vi "Actor Core.vi"(8 "error in":errorcluster, 11 "Nested in":refnum<class "UI Actor.lvclass">) -> (0 "error out":errorcluster, 3 "Actor out":refnum<class "Actor.lvclass">)   [LabVIEW 2020, in "UI Actor.lvlib" / "UI Actor.lvclass"]
doc: "(<B>Filename</B>: Actor Framework.lvlib:Actor.lvclass:Actor Core.vi)\n\nReceives messages to the actor, reacts to them, and initiates any error handling that may shut the actor down.\n\nDescendant classes may override this VI to append parallel tasks for the actor to complete while it handles messages. Overrides use the Call Parent Method node."
uses:
  UI Actor.lvclass
  C:/Program Files (x86)/National Instruments/LabVIEW 2020/vi.lib/ActorFramework/Actor/Actor.lvclass
  <vilib>/ActorFramework/Actor/Actor.lvclass
  <vilib>/ActorFramework/Actor/Actor.lvclass/Actor.ctl
  <vilib>/ActorFramework/Message Enqueuer/Message Enqueuer.lvclass/Message Enqueuer.ctl
  UI Actor.lvclass/UI Actor.ctl
  UI Actor Messages/Read ADC Msg/Read ADC Msg.lvclass/Read ADC Msg.ctl
  UI Actor Messages/Set Pin Status Msg/Set Pin Status Msg.lvclass/Set Pin Status Msg.ctl
  <vilib>/ActorFramework/Message Enqueuer/Init from Existing Queue.vi
  <vilib>/ActorFramework/Message Enqueuer/Enqueue.vi
  <vilib>/ActorFramework/Stop Msg/Stop Msg.lvclass
  C:/Program Files (x86)/National Instruments/LabVIEW 2020/vi.lib/ActorFramework/Message/Message.lvclass
  UI Actor Messages/Read ADC Msg/Read ADC Msg.lvclass
  UI Actor Messages/Set Pin Status Msg/Set Pin Status Msg.lvclass
  <vilib>/ActorFramework/Message Priority Queue/Priority Enqueue.vi
  <vilib>/ActorFramework/Message Enqueuer/Message Enqueuer.lvclass
  UI Actor Messages/Set Port Status Msg/Set Port Status Msg.lvclass
panel:
  out "Port Leds":bool[](array[boolean])
  in  "Port Value":string
  in  "Set Port Status":bool
  in  "Port":string(combo)
  out "Boolean 8":bool
  out "Boolean 7":bool
  out "Boolean 6":bool
  out "Boolean 5":bool
  out "Boolean 4":bool
  out "Boolean 3":bool
  out "Boolean 2":bool
  out "Boolean":bool
  out "Array":bool[](array[boolean])
  in  "Value":string(combo)
  in  "Set Pin Status":bool
  in  "Pin LED":string(combo)
  in  "Canal LED":string(combo)
  out "TERMINAL READING":string
  in  "Canal ADC":string(combo)
  in  "Read ADC":bool
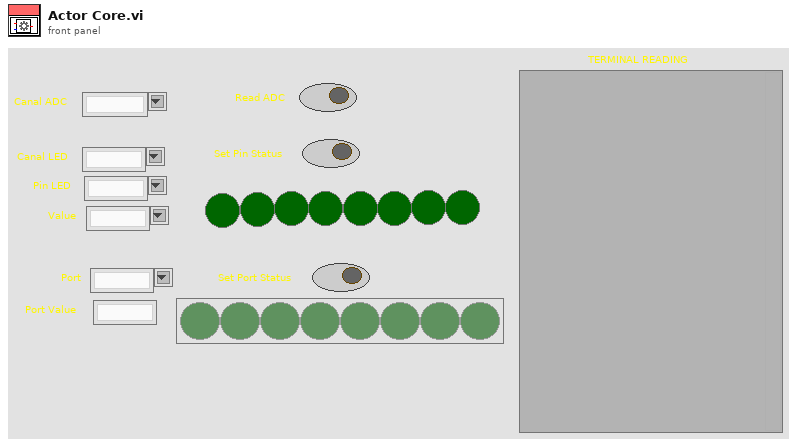
[diagram p1: front panel]
types:
  T1 = cluster{"Stop":refnum<user-event>, "TERMINAL READING":refnum<user-event>, "Array":refnum<user-event>, "Boolean 2":refnum<user-event>, "Boolean 3":refnum<user-event>, "Boolean 6":refnum<user-event>, "Boolean 8":refnum<user-event>, "Boolean 4":refnum<user-event>, "Boolean":refnum<user-event>, "Boolean 5":refnum<user-event>, "Boolean 7":refnum<user-event>, "Port Leds":refnum<user-event>}
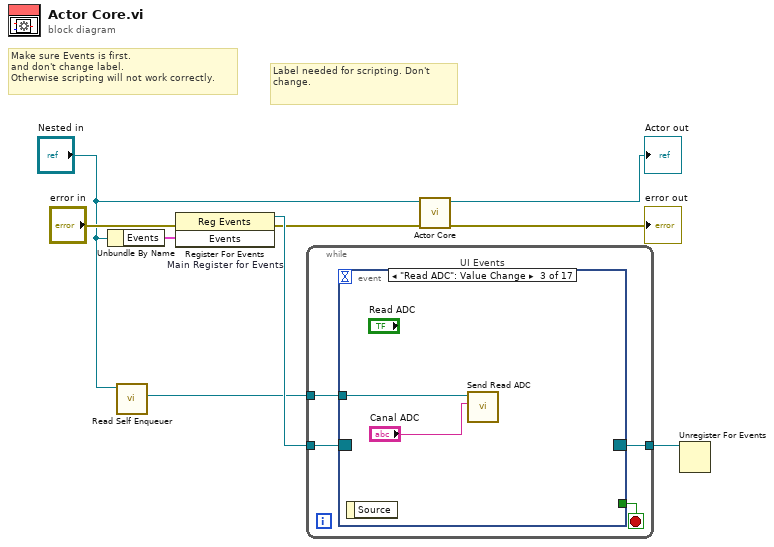
[diagram p0: block diagram]
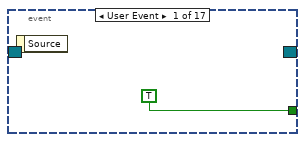
[diagram p2: hidden frame]
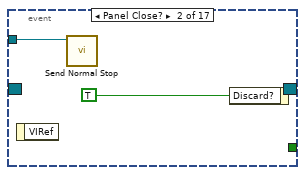
[diagram p3: hidden frame]
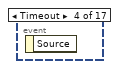
[diagram p4: hidden frame]
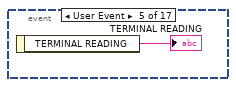
[diagram p5: hidden frame]
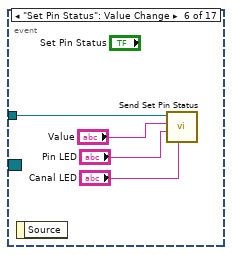
[diagram p6: hidden frame]
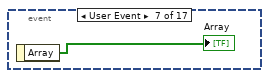
[diagram p7: hidden frame]
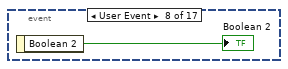
[diagram p8: hidden frame]
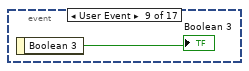
[diagram p9: hidden frame]
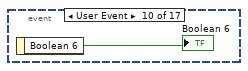
[diagram p10: hidden frame]
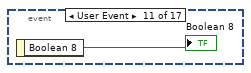
[diagram p11: hidden frame]
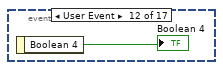
[diagram p12: hidden frame]
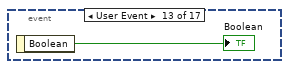
[diagram p13: hidden frame]
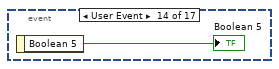
[diagram p14: hidden frame]
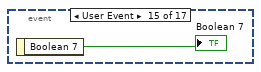
[diagram p15: hidden frame]
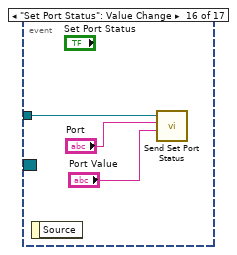
[diagram p16: hidden frame]
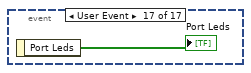
[diagram p17: hidden frame]
diagram:
  # "Label needed for scripting. Don't change."
  # "Make sure Events is first.\nand don't change label.\nOtherwise scripting will not work correctly."
  n1 = Unbundle By Name("Nested in") -> ("Events"=w6:T1)
  n2 = call <vilib>:"Read Self Enqueuer.vi"("Actor"="Nested in") -> ("Self Enqueuer"=w4:refnum<class "Message Enqueuer.lvclass">)  [unwired: 10 in]
  n3 = register-events "Main Register for Events"(error in="error in", w6) -> (reference out=w7:refnum<event-registration>, error out=w2:errorcluster)  [unwired: 1 in]
  n4 = while {
    tunnel: w7 -> [w13]
    tunnel: [w11] -> w5
    tunnel: w4 -> [w10]
    stop <- w12 stop-if-true
    n5 = event "UI Events" shown="[2] \"Read ADC\": Value Change" {
      selector: w13 -> [_ _ _ _ _ _ _ _ _ _ _ _ _ _ _ _ _]
      dyn-events: [_ _ _ _ _ _ _ _ _ _ _ _ _ _ _ _ _] -> w11
      timeout: _ -> [_ _ _ _ _ _ _ _ _ _ _ _ _ _ _ _ _]
      tunnel: [TRUE _ _ _ _ _ _ _ _ _ _ _ _ _ _ _ _] -> w12
      tunnel: w10 -> [_ w15 w18 _ _ w23 _ _ _ _ _ _ _ _ _ w35 _]
      event User Event {
        n6 = event-data() -> ()  [unwired: 1 in, 1 out]
      }
      event Panel Close? {
        n7 = event-data() -> ()  [unwired: 1 in, 1 out]
        n8 = call <vilib>:"Send Normal Stop.vi"("Message Enqueuer"=w15) -> ()  [unwired: 10 in, 1 out]
        n9 = event-data("Discard?"=TRUE) -> ()  [unwired: 1 in, 1 out]
      }
      event "Read ADC": Value Change {
        n10 = event-data() -> ()  [unwired: 1 in, 1 out]
        n11 = call "Send Read ADC.vi"("Canal"="Canal ADC", "Message Enqueuer"=w18) -> ()  [unwired: 8 in, 2 out]
      }
      event Timeout {
        n12 = event-data() -> ()  [unwired: 1 in, 1 out]
      }
      event User Event {
        n13 = event-data() -> ("TERMINAL READING"=→"TERMINAL READING":string)  [unwired: 1 in]
      }
      event "Set Pin Status": Value Change {
        n14 = event-data() -> ()  [unwired: 1 in, 1 out]
        n15 = call "Send Set Pin Status.vi"("Puerto"="Canal LED", "Pin"="Pin LED", "Valor"="Value", "Message Enqueuer"=w23) -> ()  [unwired: 6 in, 2 out]
      }
      event User Event {
        n16 = event-data() -> ("Array"=→"Array":bool[])  [unwired: 1 in]
      }
      event User Event {
        n17 = event-data() -> ("Boolean 2"=→"Boolean 2":bool)  [unwired: 1 in]
      }
      event User Event {
        n18 = event-data() -> ("Boolean 3"=→"Boolean 3":bool)  [unwired: 1 in]
      }
      event User Event {
        n19 = event-data() -> ("Boolean 6"=→"Boolean 6":bool)  [unwired: 1 in]
      }
      event User Event {
        n20 = event-data() -> ("Boolean 8"=→"Boolean 8":bool)  [unwired: 1 in]
      }
      event User Event {
        n21 = event-data() -> ("Boolean 4"=→"Boolean 4":bool)  [unwired: 1 in]
      }
      event User Event {
        n22 = event-data() -> ("Boolean"=→"Boolean":bool)  [unwired: 1 in]
      }
      event User Event {
        n23 = event-data() -> ("Boolean 5"=→"Boolean 5":bool)  [unwired: 1 in]
      }
      event User Event {
        n24 = event-data() -> ("Boolean 7"=→"Boolean 7":bool)  [unwired: 1 in]
      }
      event "Set Port Status": Value Change {
        n25 = event-data() -> ()  [unwired: 1 in, 1 out]
        n26 = call "Send Set Port Status.vi"("Valor HEX"="Port Value", "Puerto"="Port", "Message Enqueuer"=w35) -> ()  [unwired: 7 in, 2 out]
      }
      event User Event {
        n27 = event-data() -> ("Port Leds"=→"Port Leds":bool[])  [unwired: 1 in]
      }
    }
  }
  n28 = call-parent "Actor Core.vi"("error in"=w2, "Actor in"="Nested in") -> ("error out"=→"error out":errorcluster, "Actor out"=→"Actor out":refnum<class "Actor.lvclass">)  [unwired: 8 in]
  n29 = Unregister For Events(event registration refnum=w5) -> ()  [unwired: 1 in, 1 out]
